vi "set channel property caen.vi"(0 "VISA in":refnum<visa-resource-name>, 5 "Value":variant, 7 "Channel":T1={" Card.Channel"=1.12, "Crate"=0} {"Card.Channel" format="%.2f"}, 9 "Property":T2, 11 "error in":errorcluster) -> (4 "VISA out":refnum<visa-resource-name>, 15 "error out":errorcluster)   [LabVIEW 2018]
uses:
  Channel Properties.ctl
  channel.ctl
  set location.ctl
  CAEN globals.vi
  <vilib>/regexp/Match Regular Expression.xnode
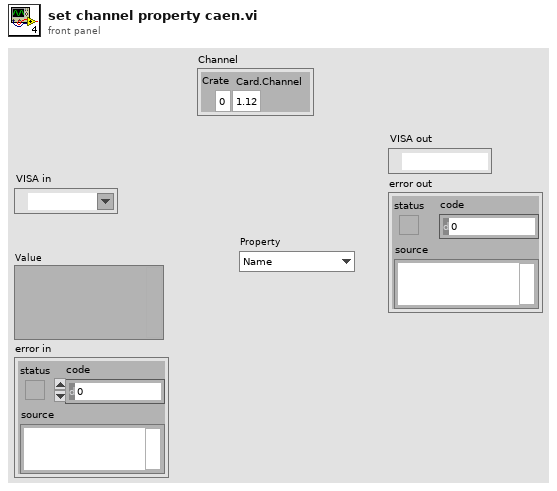
[diagram p1: front panel]
types:
  T1 = typedef "channel.ctl" = cluster{" Card.Channel":dbl, "Crate":i32}
  T2 = typedef "Channel Properties.ctl" = enum16{"Name", "Vset", "Vfile", "Vswmax", "Iset", "Enable", "Flag", "Vbackup"}
  T3 = typedef "location cluster.ctl" = cluster{"Column":i32, "Card Type":string, "Channel":i32, "Card":i32, "Default response":string, "Entering":string, "Entering state":bool, "subpage":i32, "page":i32, "Crate":i32, "Screen":string, "Group":string, "Global HV Enable":bool, "Vsel_buffer":bool, "Vdisp_buffer":bool}
  T4 = cluster{"Group Name":string, "Channels in Group":T1[]}[]
  T5 = typedef "crate.ctl" = cluster{"CAENet Address":i32, "Crate Model":string, "Firmware Version":string, "Crate Map":T6[], "Total Channels":i32}
  T6 = typedef "card.ctl" = cluster{"Slot Number":i32, "Card Model":string, "Num Channels":i32, "Polarity":string, "Vmax":dbl, "Imax":dbl, "Revision":string}
  T7 = typedef "set location.ctl" = cluster{"set index":i32, "set Screen":string, "set subpage":i32, "set column":i32, "Group":string, "Crate":i32}
  T8 = typedef "channel_cluster.ctl" = cluster{"Channel Name":string, "Crate":i32, "Card Type":string, "Card":i32, "Channel":i32, "Status Icon":picture, "Vmon (V)":dbl, "Vset (V)":dbl, "Imon (A)":dbl, "Iset (A)":dbl, "Timestamp":string, "ON/OFF":bool, "Status":string, "Vswmax (V)":dbl, "Flag":bool, "Vfile (V)":dbl, "Error Logged":bool[], "enable_file":bool}
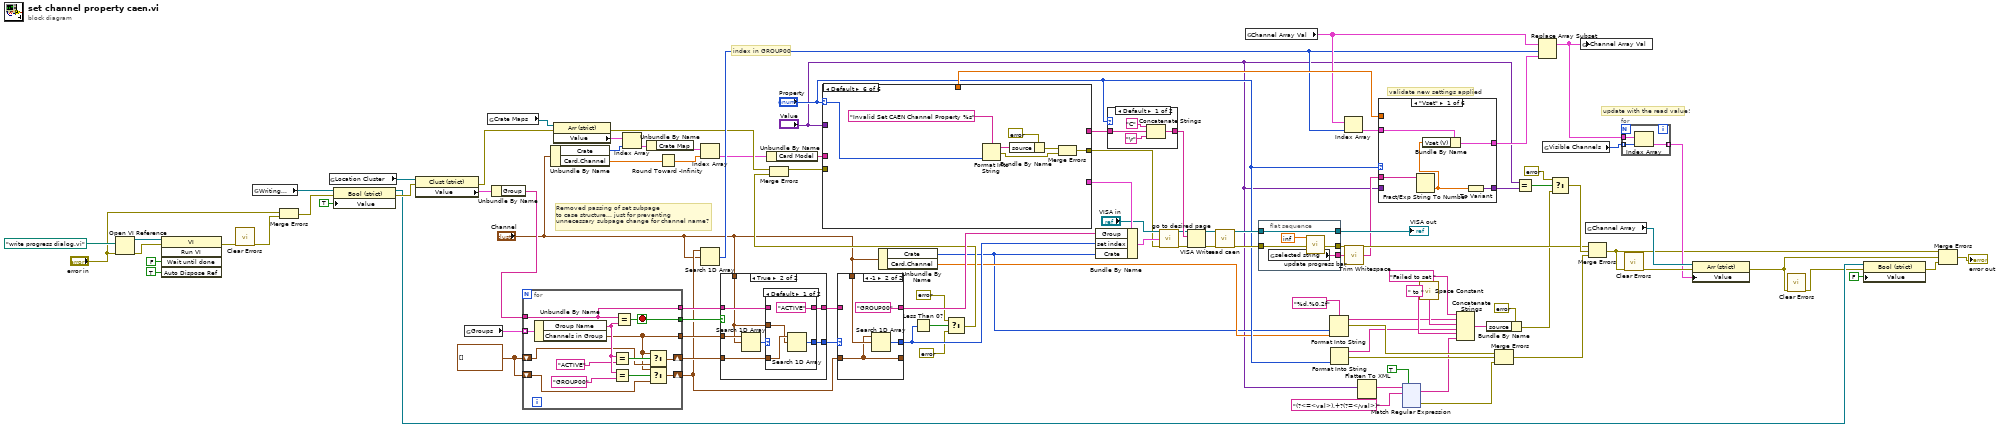
[diagram p0: block diagram]
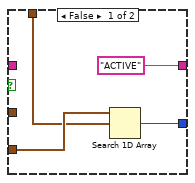
[diagram p4: hidden frame]
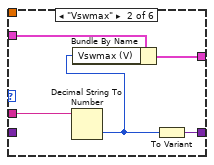
[diagram p6: hidden frame]
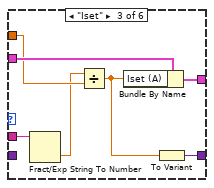
[diagram p7: hidden frame]
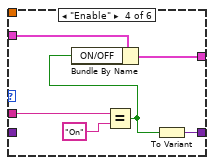
[diagram p8: hidden frame]
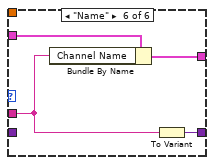
[diagram p10: hidden frame]
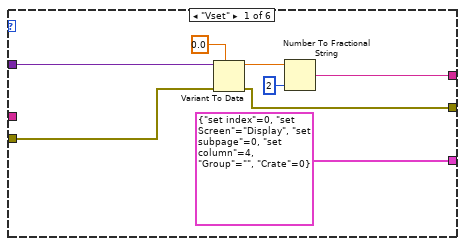
[diagram p11: hidden frame]
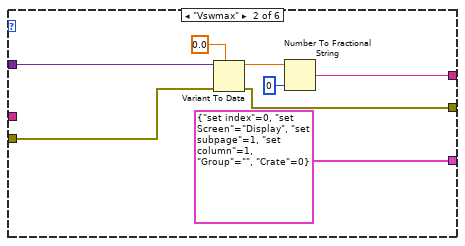
[diagram p12: hidden frame]
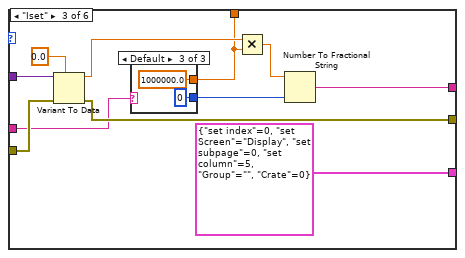
[diagram p13: hidden frame]
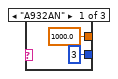
[diagram p14: hidden frame]
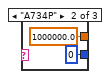
[diagram p15: hidden frame]
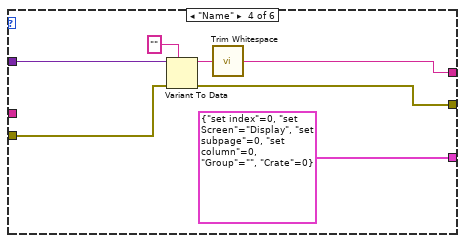
[diagram p16: hidden frame]
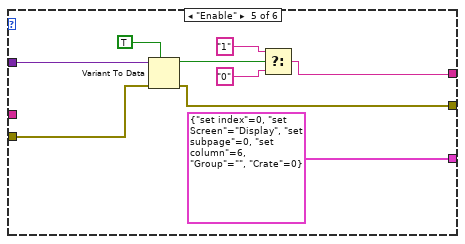
[diagram p17: hidden frame]
diagram:
  w21 = T1[] [] ("Channels in Group")
  # "Removed passing of set subpage\nto case structure... just for preventing\nunnecessary subpage change for channel name?"
  # "index in GROUP00"
  # "update with the read value!"
  # "validate new settings applied"
  n1 = Open VI Reference(vi path=path "write progress dialog.vi", error in (no error)="error in") -> (vi reference=w49:refnum<vi>, error out=w48:errorcluster)  [unwired: 4 in]
  n2 = invoke class="VI" method="Run VI"(reference=w49, error in=w48, "Wait until done"=FALSE ("Wait Until Done"), "Auto Dispose Ref"=TRUE ("Auto Dispose Reference")) -> (error out=w45:errorcluster)  [unwired: 1 in, 4 out]
  n3 = call <vilib>:"Clear Errors.vi"("error in (no error)"=w45) -> ("error out"=w43:errorcluster)  [unwired: 5 in, 1 out]
  n4 = global read "CAEN globals.vi" "Writing..."() -> (w81:refnum<vi>)
  n5 = Merge Errors("error in", w43) -> (w44:errorcluster)
  n6 = global read "CAEN globals.vi" "Location Cluster"() -> (w86:refnum<vi>)
  n7 = property class="Bool (strict)"(reference=w81, error in=w44, "Value"=TRUE) -> (reference out=w77:refnum<vi>, error out=w80:errorcluster)
  n8 = property class="Clust (strict)"(reference=w86, error in=w80) -> (error out=w12:errorcluster, "Value"=w85:T3)  [unwired: 1 out]
  n9 = global read "CAEN globals.vi" "Groups"() -> (w76:T4)
  n10 = global read "CAEN globals.vi" "Crate Maps"() -> (w18:refnum<vi>)
  n11 = Unbundle By Name(w85) -> ("Group"=w20:string)
  n12 = for {
    tunnel: w76 -> [w113] mode=indexing
    tunnel: w20 -> [w111]
    tunnel: [w112] -> w84
    tunnel: [w101] -> w83
    tunnel: [w111] -> w82
    shift-right: [w103] -> w22
    shift-left: w21 -> [w102]
    shift-right: [w105] -> w19
    shift-left: w21 -> [w104]
    stop <- w112 stop-if-true
    n13 = Unbundle By Name(w113) -> ("Group Name"=w110:string, "Channels in Group"=w101:T1[])
    n14 = Equal?(x=w110, y="ACTIVE" ("Group")) -> (x = y?=w107:bool)
    n15 = Equal?(x=w110, y="GROUP00" ("Group")) -> (x = y?=w106:bool)
    n16 = Equal?(x=w111, y=w110) -> (x = y?=w112:bool)
    n17 = Select(t=w101, s=w107, f=w102) -> (s? t:f=w103:T1[])
    n18 = Select(t=w101, s=w106, f=w104) -> (s? t:f=w105:T1[])
  }
  n19 = Unbundle By Name("Channel") -> ("Crate"=w6:i32, "Card.Channel"=w5:dbl)
  n20 = property class="Arr (strict)"(reference=w18, error in=w12) -> (error out=w11:errorcluster, "Value"=w17:T5[])  [unwired: 1 out]
  n21 = Index Array(array=w17, index=w6) -> (element=w16:T5)
  n22 = Unbundle By Name(w16) -> ("Crate Map"=w14:T6[])
  n23 = Round Toward -Infinity(1:w5) -> (0:w13:dbl)
  n24 = Index Array(array=w14, index=w13) -> (element=w10:T6)
  n25 = Search 1D Array(1D array=w19, element="Channel") -> (index of element=w63:i32)  [unwired: 1 in]
  n26 = case shown="True" w84 {
    tunnel: "Channel" -> [w115 w118]
    tunnel: w83 -> [_ w124]
    tunnel: [w114 w122] -> w58
    tunnel: ["ACTIVE" ("Group") w121] -> w56
    tunnel: w82 -> [_ w120]
    tunnel: w22 -> [w116 w119]
    frame False {
      n27 = Search 1D Array(1D array=w116, element=w115) -> (index of element=w114:i32)  [unwired: 1 in]
    }
    frame True {
      n28 = Search 1D Array(1D array=w124, element=w118) -> (index of element=w123:i32)  [unwired: 1 in]
      n29 = case shown="Default" w123 {
        selector: w123 -> [_ w130]
        tunnel: [w127 w130] -> w122
        tunnel: ["ACTIVE" ("Group") w129] -> w121
        tunnel: w120 -> [_ w129]
        tunnel: w119 -> [w126 _]
        tunnel: w118 -> [w125 _]
        frame Default {
          n30 = Search 1D Array(1D array=w126, element=w125) -> (index of element=w127:i32)  [unwired: 1 in]
        }
        frame 0.. {
        }
      }
    }
  }
  n31 = Unbundle By Name(w10) -> ("Card Model"=w9:string)
  n32 = case shown="Default" "Property" {
    selector: "Property" -> [_ _ _ _ _ w181]
    tunnel: [T7 {"set index"=0, "set Screen"="Display", "set subpage"=0, "set column"=4, "Group"="", "Crate"=0} ("Set Cluster") T7 {"set index"=0, "set Screen"="Display", "set subpage"=1, "set column"=1, "Group"="", "Crate"=0} ("Set Cluster") T7 {"set index"=0, "set Screen"="Display", "set subpage"=0, "set column"=5, "Group"="", "Crate"=0} ("Set Cluster") T7 {"set index"=0, "set Screen"="Display", "set subpage"=0, "set column"=0, "Group"="", "Crate"=0} ("Set Cluster") T7 {"set index"=0, "set Screen"="Display", "set subpage"=0, "set column"=6, "Group"="", "Crate"=0} ("Set Cluster") _] -> w96
    tunnel: [w135 w143 w156 w165 w171 _] -> w93
    tunnel: "Value" -> [w133 w141 w154 w169 w177 _]
    tunnel: [w132 w140 w153 w164 w175 w182] -> w89
    tunnel: w11 -> [w131 w139 w152 w168 w176 _]
    tunnel: [_ _ w148 _ _ _] -> w66
    tunnel: w9 -> [_ _ w147 _ _ _]
    frame "Vset" {
      n33 = Variant To Data(error in=w131, type=0.0 ("precision (6)"), Variant=w133) -> (data=w137:dbl, error out=w132:errorcluster)
      n34 = Number To Fractional String(number=w137, precision (6)=i16 2) -> (F-format string=w135:string)  [unwired: 2 in]
    }
    frame "Vswmax" {
      n35 = Variant To Data(error in=w139, type=0.0 ("precision (6)"), Variant=w141) -> (data=w145:dbl, error out=w140:errorcluster)
      n36 = Number To Fractional String(number=w145, precision (6)=i16 0) -> (F-format string=w143:string)  [unwired: 2 in]
    }
    frame "Iset" {
      n37 = Variant To Data(error in=w152, type=0.0 ("precision (6)"), Variant=w154) -> (data=w150:dbl, error out=w153:errorcluster)
      n38 = case shown="Default" w147 {
        tunnel: [i16 3 ("precision (6)") i16 0 ("precision (6)") i16 0 ("precision (6)")] -> w151
        tunnel: [1000.0 ("precision (6)") 1000000.0 ("precision (6)") 1000000.0 ("precision (6)")] -> w148
        frame "A932AN" {
        }
        frame "A734P" {
        }
        frame Default {
        }
      }
      n39 = Multiply(x=w150, y=w148) -> (x*y=w149:dbl)
      n40 = Number To Fractional String(number=w149, precision (6)=w151) -> (F-format string=w156:string)  [unwired: 2 in]
    }
    frame "Name" {
      n41 = Variant To Data(error in=w168, type="" ("string"), Variant=w169) -> (data=w167:string, error out=w164:errorcluster)
      n42 = call <vilib>:"Trim Whitespace.vi"("string"=w167) -> ("trimmed string"=w165:string)  [unwired: 1 in]
    }
    frame "Enable" {
      n43 = Variant To Data(error in=w176, type=TRUE ("status"), Variant=w177) -> (data=w174:bool, error out=w175:errorcluster)
      n44 = Select(t="1" ("Group"), s=w174, f="0" ("Group")) -> (s? t:f=w171:string)
    }
    frame Default {
      n45 = Format Into String(format string="Invalid Set CAEN Channel Property %s" ("source"), w181) -> (resulting string=w184:string, error out=w180:errorcluster)  [unwired: 2 in]
      n46 = Bundle By Name(cluster=errorcluster {"status"=TRUE, "code"=0, "source"=""} ("error out 2"), "source"=w184) -> (w183:errorcluster)
      n47 = Merge Errors(w183, w180) -> (w182:errorcluster)
    }
  }
  n48 = case shown="-1" w58 {
    selector: w58 -> [w188 _]
    tunnel: "Channel" -> [_ w191]
    tunnel: [w188 w193] -> w55
    tunnel: [w189 "GROUP00" ("Group")] -> w57
    tunnel: w56 -> [w189 _]
    tunnel: w19 -> [w187 w190]
    tunnel: [w187 w190] -> _
    frame Default {
    }
    frame -1 {
      n49 = Search 1D Array(1D array=w190, element=w191) -> (index of element=w193:i32)  [unwired: 1 in]
    }
  }
  n50 = Unbundle By Name("Channel") -> ("Crate"=w7:i32, "Card.Channel"=w8:dbl)
  n51 = Less Than 0?(x=w55) -> (x < 0?=w54:bool)
  n52 = Select(t=errorcluster {"status"=TRUE, "code"=0, "source"="Channel not found"} ("error out"), s=w54, f=errorcluster {"status"=FALSE, "code"=0, "source"=""} ("error out")) -> (s? t:f=w51:errorcluster)
  n53 = Merge Errors(w11, w51) -> ()  [unwired: 1 out]
  n54 = Bundle By Name(cluster=w96, "Group"=w57, "set index"=w55, "Crate"=w7) -> (w100:T7)
  n55 = case shown="Default" "Property" {
    tunnel: [w195 w198] -> w97
    tunnel: w93 -> [w194 w198]
    frame Default {
      n56 = Concatenate Strings("C" ("string"), w194, "\r" ("string")) -> (w195:string)
    }
    frame "Enable" {
    }
  }
  n57 = call "go to desired page.vi"("VISA in"="VISA in", "Set Cluster"=w100, "error in"=w89) -> ("VISA out"=w95:refnum<visa-resource-name>, "error out"=w94:errorcluster)  [unwired: 9 in, 2 out]
  n58 = VISA Write(VISA resource name=w95, write buffer=w97, error in (no error)=w94) -> (VISA resource name out=w99:refnum<visa-resource-name>, error out=w98:errorcluster)  [unwired: 1 out]
  n59 = call "read caen.vi"("VISA in"=w99, "error in"=w98) -> ("VISA out"=w75:refnum<visa-resource-name>, "error out"=w68:errorcluster)  [unwired: 8 in, 4 out]
  n60 = global read "CAEN globals.vi" "Channel Array Val"() -> (w64:T8[])
  n61 = flat-sequence {
    tunnel: [w202] -> w91
    tunnel: w75 -> [w202]
    tunnel: w68 -> [w201]
    tunnel: [w201] -> w72
    tunnel: [w200] -> w70
    frame #0 {
      n62 = global read "CAEN globals.vi" "selected string"() -> (w200:string)
      n63 = call "update progress bar.vi"("Progress"=inf) -> ()  [unwired: 6 in, 1 out]
    }
  }
  n64 = Format Into String(format string="%d.%0.2f", w7, w8) -> (resulting string=w34:string, error out=w31:errorcluster)  [unwired: 2 in]
  n65 = Format Into String("Property") -> (resulting string=w29:string, error out=w30:errorcluster)  [unwired: 3 in]
  n66 = Index Array(array=w64, index=w63) -> (element=w69:T8)
  n67 = call <vilib>:"Trim Whitespace.vi"("string"=w70) -> ("trimmed string"=w71:string)  [unwired: 1 in]
  n68 = Flatten To XML(anything="Value") -> (xml string=w27:string)
  n69 = case shown="\"Vset\"" "Property" {
    tunnel: w71 -> [w206 w211 w218 w224 _ w229]
    tunnel: [w207 w212 w219 w225 w226 w231] -> w90
    tunnel: w69 -> [w205 w210 w217 w222 w227 w230]
    tunnel: [w203 w208 w216 w221 w227 w228] -> w65
    tunnel: w66 -> [_ _ w215 _ _ _]
    tunnel: "Value" -> [_ _ _ _ w226 _]
    frame "Vset" {
      n70 = Fract/Exp String To Number(string=w206) -> (number=w204:dbl)  [unwired: 3 in, 1 out]
      n71 = Bundle By Name(cluster=w205, "Vset (V)"=w204) -> (w203:T8)
      n72 = To Variant(anything=w204) -> (Variant=w207:variant)
    }
    frame "Vswmax" {
      n73 = Decimal String To Number(string=w211) -> (number=w209:i32)  [unwired: 2 in, 1 out]
      n74 = Bundle By Name(cluster=w210, "Vswmax (V)"=w209) -> (w208:T8)
      n75 = To Variant(anything=w209) -> (Variant=w212:variant)
    }
    frame "Iset" {
      n76 = Fract/Exp String To Number(string=w218) -> (number=w214:dbl)  [unwired: 3 in, 1 out]
      n77 = Divide(x=w214, y=w215) -> (x/y=w213:dbl)
      n78 = Bundle By Name(cluster=w217, "Iset (A)"=w213) -> (w216:T8)
      n79 = To Variant(anything=w213) -> (Variant=w219:variant)
    }
    frame "Enable" {
      n80 = Equal?(x=w224, y="On" ("x")) -> (x = y?=w220:bool)
      n81 = Bundle By Name(cluster=w222, "ON/OFF"=w220) -> (w221:T8)
      n82 = To Variant(anything=w220) -> (Variant=w225:variant)
    }
    frame Default {
      # "channel property\nnot applicable"
    }
    frame "Name" {
      n83 = Bundle By Name(cluster=w230, "Channel Name"=w229) -> (w228:T8)
      n84 = To Variant(anything=w229) -> (Variant=w231:variant)
    }
  }
  n85 = xnode "Match Regular Expression"("input string"=w27, "regular expression"="(?<=<val>).+?(?=</val>)" ("xml string"), "ignore case? (F)"=TRUE) -> ("whole match"=w24:string, "error out"=w23:errorcluster)  [unwired: 3 in, 3 out]
  n86 = call <vilib>:"Space Constant.vi"() -> ("String"=w38:string)
  n87 = Concatenate Strings("Failed to set " ("source"), w34, w38, w29, " to " ("string"), w24) -> (w40:string)
  n88 = Bundle By Name(cluster=errorcluster {"status"=TRUE, "code"=0, "source"="Value not set"} ("error in"), "source"=w40) -> (w35:errorcluster)
  n89 = Merge Errors(w31, w30, w23) -> (w32:errorcluster)
  n90 = Equal?(x="Value", y=w90) -> (x = y?=w88:bool)
  n91 = Replace Array Subset(array=w64, new element=w65, index=w63) -> (w62:T8[])
  n92 = global read "CAEN globals.vi" "Visible Channels"() -> (w61:i32[])
  n93 = Select(t=errorcluster {"status"=FALSE, "code"=0, "source"=""} ("error in"), s=w88, f=w35) -> (s? t:f=w87:errorcluster)
  n94 = global write "CAEN globals.vi" "Channel Array Val"(w62) -> ()
  n95 = global read "CAEN globals.vi" "Channel Array"() -> (w60:refnum<vi>)
  n96 = Merge Errors(w72, w87, w32) -> (w3:errorcluster)
  n97 = for {
    tunnel: w62 -> [w234]
    tunnel: w61 -> [w233] mode=indexing
    tunnel: [w232] -> w59 mode=indexing
    n98 = Index Array(array=w234, index=w233) -> (element=w232:T8)
  }
  n99 = call <vilib>:"Clear Errors.vi"("error in (no error)"=w3) -> ("error out"=w67:errorcluster)  [unwired: 5 in, 1 out]
  n100 = property class="Arr (strict)"(reference=w60, error in=w67, "Value"=w59) -> (error out=w2:errorcluster)  [unwired: 1 out]
  n101 = call <vilib>:"Clear Errors.vi"("error in (no error)"=w2) -> ("error out"=w1:errorcluster)  [unwired: 5 in, 1 out]
  n102 = property class="Bool (strict)"(reference=w77, error in=w1, "Value"=FALSE) -> (error out=w74:errorcluster)  [unwired: 1 out]
  n103 = Merge Errors(w3, w2, w74) -> (→"error out":errorcluster)
  "VISA out" <- w91
